vi "Version.vi"() -> ()   [LabVIEW 2014]
panel:
  in  "布尔":bool=TRUE
  # "XXXXXXXXXXXXXXX系统软件属"
  # "XXXXXX有限公司"
  # "禁止非法仿制硬件及拷贝软件，违者必究"
  # "电       话：027-XXXXXXXX\n传       真：027-XXXXXXXX\n网       址：XXXXXXXXXXXXXXXX\n通信地址：XXXXXXXXXXXXXXXX"
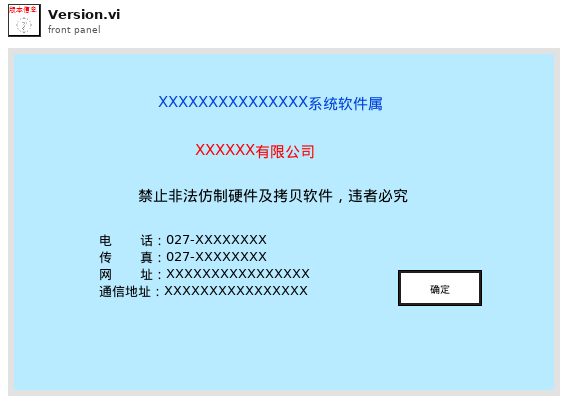
[diagram p1: front panel]
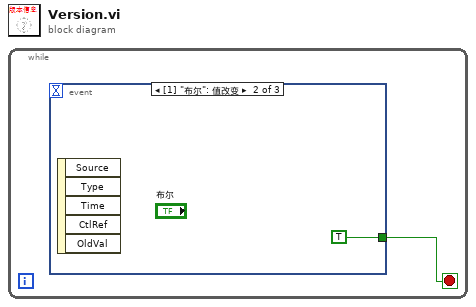
[diagram p0: block diagram]
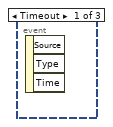
[diagram p2: hidden frame]
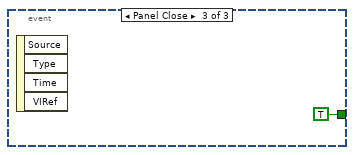
[diagram p3: hidden frame]
diagram:
  n1 = while {
    stop <- w1 stop-if-true
    n2 = event shown="[1] \"布尔\": 值改变" {
      selector: _ -> [_ _ _]
      dyn-events: _ -> [_ _ _]
      timeout: _ -> [_ _ _]
      tunnel: [_ TRUE TRUE] -> w1
      event Timeout {
        n3 = event-data() -> ()  [unwired: 1 in, 3 out]
      }
      event "布尔": Value Change {
        n4 = event-data() -> ()  [unwired: 1 in, 5 out]
      }
      event Panel Close {
        n5 = event-data() -> ()  [unwired: 1 in, 4 out]
      }
    }
  }
